vi "Initialize Actor.vi"(8 "error in (no error)":errorcluster, 11 "Actor in":refnum<class "Actor.lvclass">) -> (0 "error out":errorcluster, 3 "Actor-Interface":refnum<data-value>)   [LabVIEW 2018, in "Actor.lvlib" / "Actor-Interface.lvclass"]
uses:
  Actor-Interface.lvclass
  Actor.lvclass
  Stopped.ctl
  Events.ctl
  Stop.ctl
  Launched.ctl
  Actor-Interface.lvclass/Actor-Interface.ctl
  Event-Wrapper.lvclass
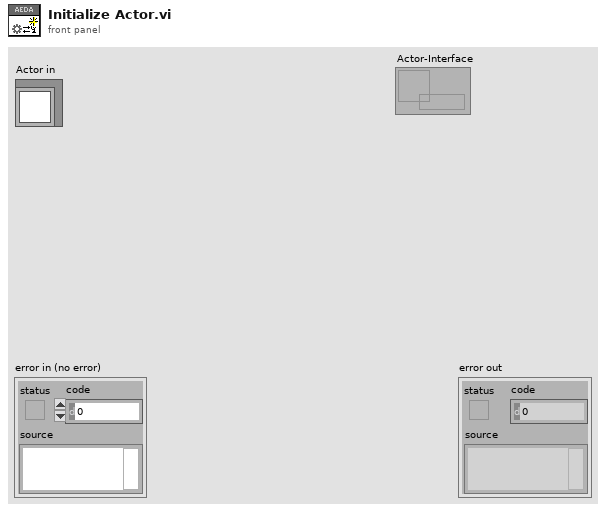
[diagram p1: front panel]
types:
  T1 = typedef "Actor.lvlib/Actor-Interface.lvclass/Events.ctl" = cluster{"Stop":refnum<user-event>, "Launched":refnum<user-event>}
  T2 = typedef "Actor.lvlib/Actor-Interface.lvclass/Stopped.ctl" = cluster{"Actor":refnum<class "Actor.lvclass">, "Final Error":errorcluster}
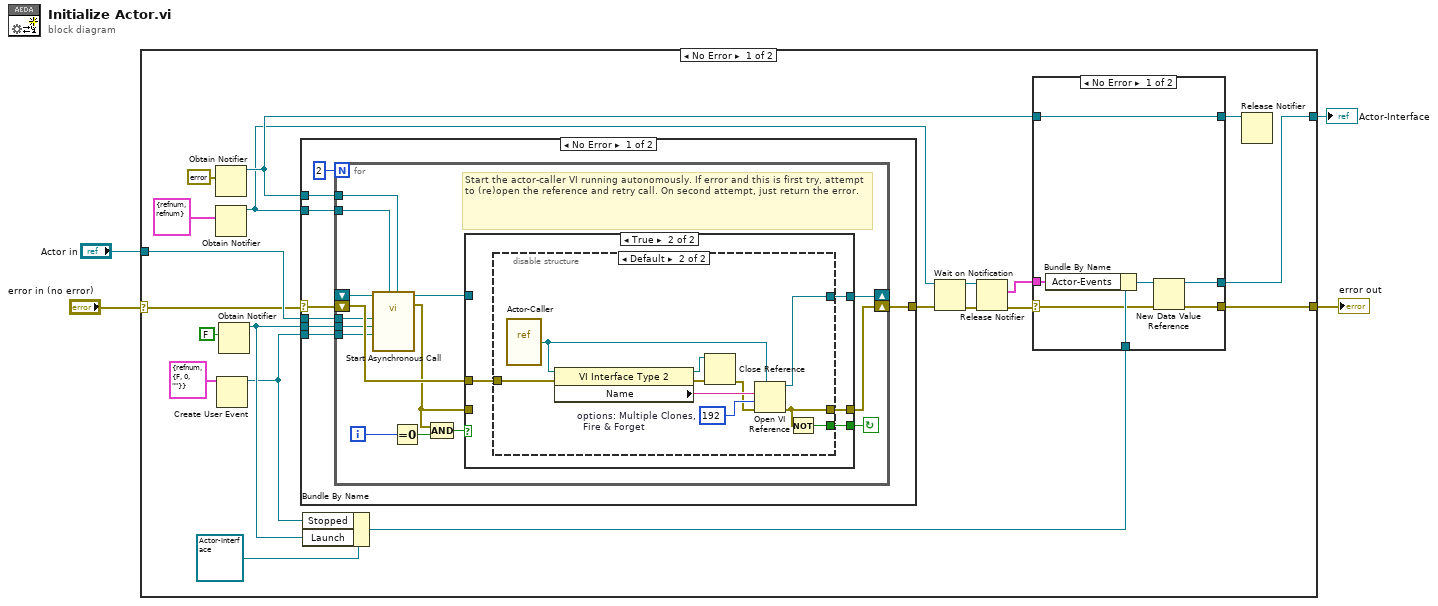
[diagram p0: block diagram]
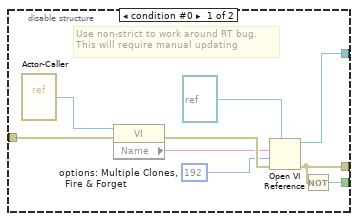
[diagram p3: hidden frame]
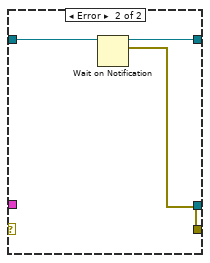
[diagram p5: hidden frame]
diagram:
  n1 = case shown="No Error" "error in (no error)" {
    selector: "error in (no error)" -> [w5 w84]
    tunnel: [w22 w84] -> w3
    tunnel: "Actor in" -> [w17 _]
    tunnel: [w21 _] -> w1
    frame No Error {
      n2 = Obtain Notifier(notification data type=errorcluster {"status"=FALSE, "code"=0, "source"=""} ("error constant")) -> (notifier out=w18:refnum<notifier>)  [unwired: 3 in, 2 out]
      n3 = Obtain Notifier(notification data type=T1 {"Stop"=refnum, "Launched"=refnum} ("Actor-Events")) -> (notifier out=w10:refnum<notifier>)  [unwired: 3 in, 2 out]
      n4 = Create User Event(user event datatype=T2 {"Actor"=refnum, "Final Error"={"status"=FALSE, "code"=0, "source"=""}} ("Stopped")) -> (user event=w14:refnum<user-event>)  [unwired: 1 in, 1 out]
      n5 = Obtain Notifier(notification data type=FALSE ("Launch")) -> (notifier out=w16:refnum<notifier>)  [unwired: 3 in, 2 out]
      n6 = case shown="No Error" w5 {
        selector: w5 -> [w30 w73]
        tunnel: [w31 w73] -> w12
        tunnel: w10 -> [w29 _]
        tunnel: w18 -> [w28 _]
        tunnel: w17 -> [w27 _]
        tunnel: w16 -> [w26 _]
        tunnel: w14 -> [w25 _]
        frame No Error {
          n7 = for {
            N: 2 -> [_]
            shift-right: [w47] -> w31
            shift-left: w30 -> [w42]
            shift-right: [w41] -> _
            shift-left: _ -> [w40]
            tunnel: w29 -> [w33]
            tunnel: w28 -> [w37]
            tunnel: w27 -> [w36]
            tunnel: w26 -> [w35]
            tunnel: w25 -> [w34]
            i -> [w44]
            stop <- w43 continue-if-true
            # "Start the actor-caller VI running autonomously. If error and this is first try, attempt to (re)open the reference and retry call. On second attempt, just return the error."
            n8 = call-by-ref "Start Asynchronous Call"(reference=w40, "Initialize-Error Passback"=w37, "Events Passback"=w33, "Stopped Event"=w34, "Launch"=w35, "Actor in"=w36) -> (reference out=w39:refnum<vi>, error out=w38:errorcluster)  [unwired: 8 in]
            n9 = Equal To 0?(x=w44) -> (x = 0?=w45:bool)
            n10 = Compound Arithmetic op=AND(w38, w45) -> (w46:bool)
            n11 = case shown="True" w46 {
              tunnel: [w48 w50] -> w41
              tunnel: [w49 w52] -> w47
              tunnel: w38 -> [w49 _]
              tunnel: [_ w53] -> w43
              tunnel: w42 -> [_ w51]
              tunnel: w39 -> [w48 _]
              frame False {
              }
              frame True {
                n12 = disable-structure shown="Default" {
                  disable-tunnel: [w59 w70] -> w53
                  disable-tunnel: [w58 w69] -> w52
                  disable-tunnel: w51 -> [w57 w68]
                  disable-tunnel: [w55 w67] -> w50
                  frame condition #0 {
                    w60 = 192  # options: Multiple Clones,   Fire & Forget
                    # "Use non-strict to work around RT bug.\nThis will require manual updating"
                    n13 = vi-ref "Actor-Caller.vi"() -> (w56:refnum<vi>)
                    n14 = property class="VI"(reference=w56, error in=w57) -> (error out=w62:errorcluster, "Name"=w61:string)  [unwired: 1 out]
                    n15 = Open VI Reference(type specifier VI Refnum (for type only)=refnum<vi> refnum, vi path=w61, options=w60, error in (no error)=w62) -> (vi reference=w55:refnum<vi>, error out=w58:errorcluster)  [unwired: 2 in]
                    n16 = Not(x=w58) -> (.not. x?=w59:bool)
                  }
                  frame condition #1 (active) {
                    w71 = 192  # options: Multiple Clones,   Fire & Forget
                    n17 = vi-ref "Actor-Caller.vi"() -> (w63:refnum<vi>)
                    n18 = property class="VI Interface Type 2"(reference=w63, error in=w68) -> (reference out=w65:refnum<vi>, error out=w66:errorcluster, "Name"=w72:string)
                    n19 = Close Reference(reference=w65, error in (no error)=w66) -> (error out=w64:errorcluster)
                    n20 = Open VI Reference(type specifier VI Refnum (for type only)=w63, vi path=w72, options=w71, error in (no error)=w64) -> (vi reference=w67:refnum<vi>, error out=w69:errorcluster)  [unwired: 2 in]
                    n21 = Not(x=w69) -> (.not. x?=w70:bool)
                  }
                }
              }
            }
          }
        }
        frame Error {
        }
      }
      n22 = Bundle By Name(cluster=refnum<class "Actor-Interface.lvclass"> refnum ("Actor.lvlib:Actor-Interface.lvclass"), "Stopped"=w14, "Launch"=w16) -> (w13:refnum<class "Actor-Interface.lvclass">)
      n23 = Wait on Notification(notifier=w10, error in (no error)=w12) -> (notifier out=w9:refnum<notifier>, error out=w8:errorcluster)  [unwired: 2 in, 2 out]
      n24 = Release Notifier(notifier=w9, error in (no error)=w8) -> (last notification=w6:T1, error out=w7:errorcluster)  [unwired: 1 in, 1 out]
      n25 = case shown="No Error" w7 {
        selector: w7 -> [w74 _]
        tunnel: w6 -> [w75 _]
        tunnel: w18 -> [w80 w83]
        tunnel: [w80 w82] -> w23
        tunnel: [w76 w81] -> w22
        tunnel: [w77 _] -> w21
        tunnel: w13 -> [w79 _]
        frame No Error {
          n26 = Bundle By Name(cluster=w79, "Actor-Events"=w75) -> (w78:refnum<class "Actor-Interface.lvclass">)
          n27 = New Data Value Reference(data value=w78, error in=w74) -> (data value reference=w77:refnum<data-value>, error out=w76:errorcluster)
        }
        frame Error {
          n28 = Wait on Notification(notifier=w83) -> (notifier out=w82:refnum<notifier>, notification=w81:errorcluster)  [unwired: 3 in, 2 out]
        }
      }
      n29 = Release Notifier(notifier=w23) -> ()  [unwired: 2 in, 3 out]
    }
    frame Error {
    }
  }
  "error out" <- w3
  "Actor-Interface" <- w1
